vi "Reachable Time Cruise.vi"(1 "Angle Displacement":dbl, 2 "Reachable Angular Velocity":dbl) -> (0 "Reachable Time Cruise":dbl)   [LabVIEW 2015]
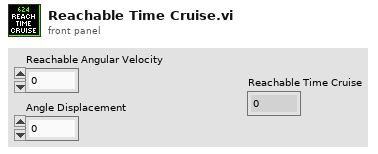
[diagram p1: front panel]
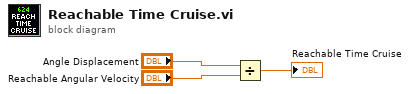
[diagram p0: block diagram]
diagram:
  n1 = Divide(x="Angle Displacement", y="Reachable Angular Velocity") -> (x/y=→"Reachable Time Cruise":dbl)
